vi "Teleop.vi"(10 "Match Info":T2={"Autonomous Elapsed Seconds"=0.0, "TeleOp Elapsed Seconds"=0.0, "Disabled Elapsed Seconds"=0.0, "Visited Autonomous"=FALSE, "Visited TeleOp"=FALSE, "Visited Disabled"=FALSE, "Autonomous Settings"={"Autonomous Style"=enum."Independent", "VI Refnum"=refnum}}, 11 "Call Context":T3) -> ()   [LabVIEW 2020]
doc: "This VI is called for each TeleOp packet received from the DS where the robot is not disabled. It is often used to read from the joysticks and update I/O or to update setpoints for timed control loops. It should complete and return within 20 milliseconds or it may miss DS packets."
uses:
  <vilib>/Rock Robotics/WPI/DriverStation/WPI_DriverStationDerivedRobotMode.ctl
  <vilib>/Rock Robotics/WPI/DriverStation/WPI_DriverStationMatch Info.ctl
  Shared Code/TypeDefs/ENUM_CMD_Mode Select.ctl
  Teleop Support/ENUM_Axes Select.ctl
  Teleop Support/ENUM_Button Select.ctl
  Systems/SwerveDrive/Cluster_CMD_ACT_Data.ctl
  Shared Code/TypeDefs/Cluster_CMD_Direction Data.ctl
  Shared Code/TypeDefs/Cluster_Module Velocity-Direction-Rotations.ctl
  Shared Code/TypeDefs/Level_Velocity plus-minus 1.ctl
  Shared Code/TypeDefs/Dial_Compase heading unit circle CCW positive.ctl
  Shared Code/TypeDefs/Cluster_X-Y.ctl
  Systems/PigeonIMU/Cluster_CMD_SEN_Data.ctl
  Systems/Tube Wheel/Cluster_CMD_ACT_Data.ctl
  Type Defs/ENUM_TubeWheel_Mode.ctl
  Type Defs/ENUM_Tube Wheel CMD Positions.ctl
  Systems/Angler/Cluster_CMD_ACT_Data.ctl
  Systems/Angler/ENUM_Input Mode.ctl
  Systems/Shooter/Cluster_CMD_ACT_Data.ctl
  Systems/Shooter/ENUM_Shooter_Mode.ctl
  Systems/Feeder/Cluster_CMD_ACT_Data.ctl
  Systems/Feeder/ENUM_CMD Mode.ctl
  Shared Code/TypeDefs/Cluster_High-Low.ctl
  8b3177bb-dc82-4863-aed5-aa104a122ccc.vi
  83fdd1ca-84e3-4cf5-86f5-8b3c56b849f5.vi
  <vilib>/Rock Robotics/Network Tables/NT Write Boolean.vi
  Systems/Game Controller/Global_SEN_Data Out.vi
  Systems/PigeonIMU/Global_CMD_SEN_Data In.vi
  Systems/Angler/Global_CMD_ACT_Data In.vi
  Systems/SwerveDrive/Global_CMD_ACT_Data In.vi
  Systems/Tube Wheel/Global_CMD_ACT_Data In.vi
  Systems/Shooter/Global_CMD_ACT_Data In.vi
  Systems/Feeder/Global_CMD_ACT_Data In.vi
  Systems/Game Controller/GameController_SEN.lvlib
  Systems/SwerveDrive/SwerveDrive_ACT_ts.lvlib
  Systems/PigeonIMU/PigeonIMU_SEN_ts.lvlib
  Systems/Tube Wheel/Tube Wheel_ACT.lvlib
  Systems/Angler/Angler_ACT.lvlib
  Systems/Shooter/Shooter_ACT.lvlib
  Systems/Feeder/Feeder_ACT.lvlib
panel:
  in  "MAx Traverse Speed FPS Out":dbl=5.0
  out "Drive Mode":T1
  out "shooter Speed Value":dbl
  in  "step value":dbl=200.0
  out "POV":i16
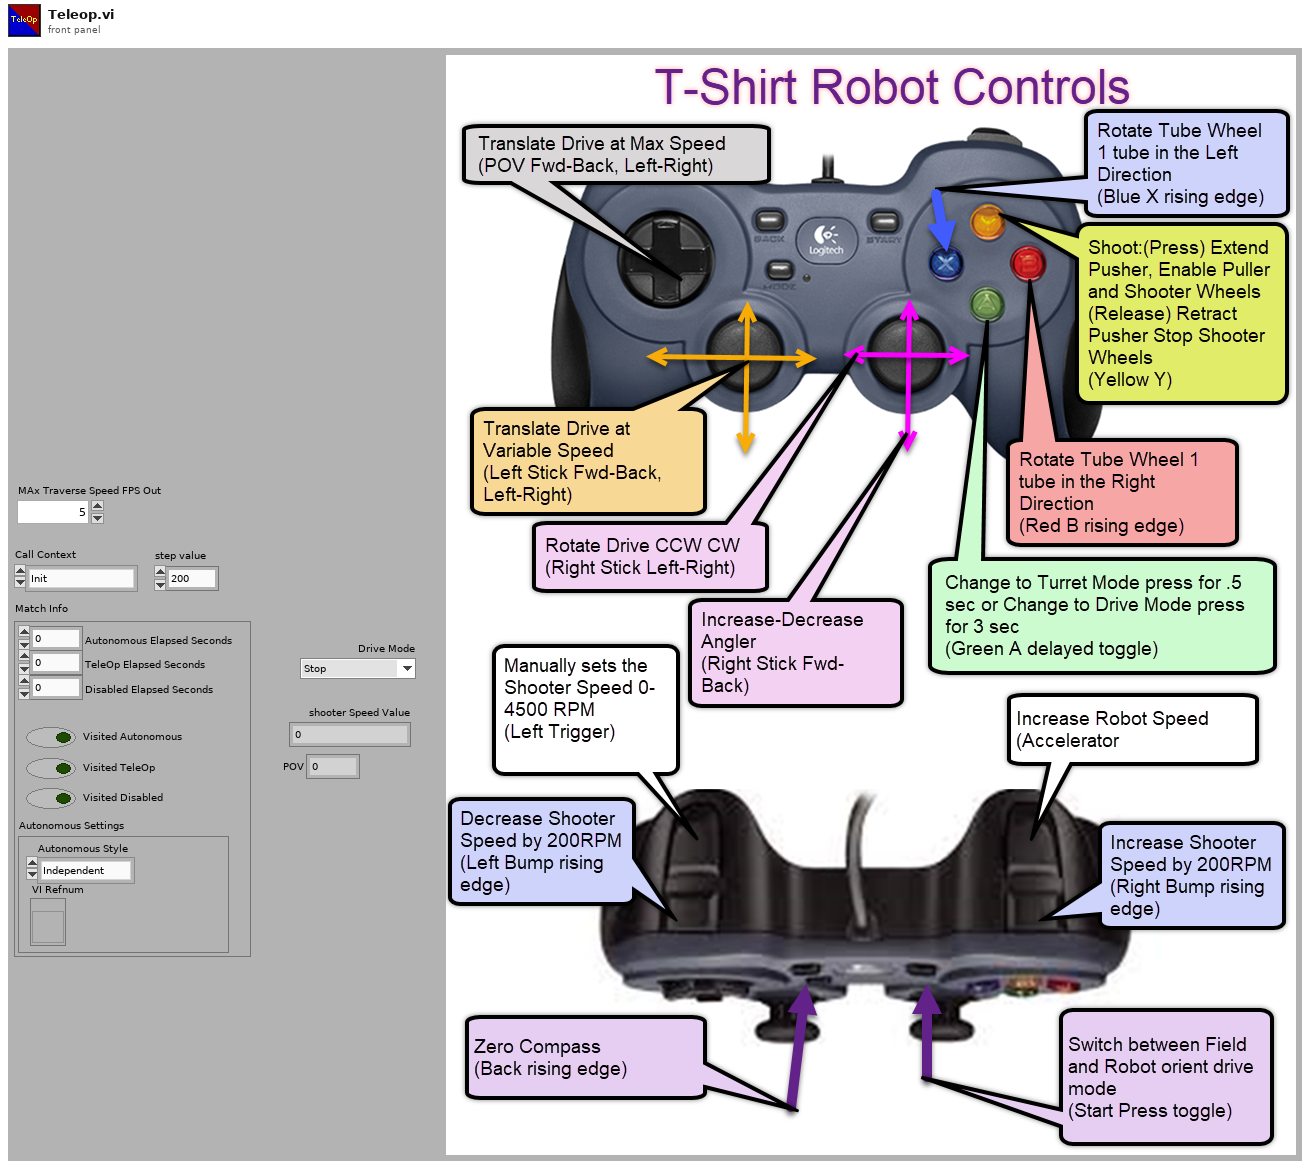
[diagram p1: front panel]
types:
  T1 = typedef "ENUM_CMD_Mode Select.ctl" = enum16{"Stop", "Move", "Turret Manual"}
  T2 = typedef "WPI_DriverStationMatch Info.ctl" = cluster{"Autonomous Elapsed Seconds":dbl, "TeleOp Elapsed Seconds":dbl, "Disabled Elapsed Seconds":dbl, "Visited Autonomous":bool, "Visited TeleOp":bool, "Visited Disabled":bool, "Autonomous Settings":cluster{"Autonomous Style":enum16{"Iterative", "Independent"}, "VI Refnum":refnum<vi>}}
  T3 = typedef "WPI_DriverStationDerivedRobotMode.ctl" = enum16{"Init", "Execute", "Stop"}
  T4 = typedef "ENUM_Axes Select.ctl" = enum16{"Left Stick Left (-1) Right (1)", "Left Stick Fwd (-1) Back(1)", "Left Trigger (0-1)", "Right Trigger (0-1)", "Right Stick Left(-1 Right (1)", "Right Stick Fwd(-1) Back (1)"}
  T5 = typedef "Cluster_High-Low.ctl" = cluster{"High":dbl, "Low":dbl}
  T6 = typedef "ENUM_Button Select.ctl" = enum16{"RightPad Green A", "RightPad Red B", "RightPad Blue X", "RightPad Yellow Y", "Left Bump", "Right Bump", "CenterPad Back", "CenterPad Start", "LeftStick Press", "RightStick Press"}
  T7 = typedef "Feeder_ACT.lvlib/Cluster_CMD_ACT_Data.ctl" = cluster{"Cmd Mode":T8, "Puller Speed (0-1":dbl}
  T8 = typedef "Feeder_ACT.lvlib/ENUM_CMD Mode.ctl" = enum16{"Stop", "Feed Pos 1", "Feed Pos 2", "Fead Full", "Back"}
  T9 = typedef "Shooter_ACT.lvlib/Cluster_CMD_ACT_Data.ctl" = cluster{"Mode":T10, "Speed Value":dbl}
  T10 = typedef "Shooter_ACT.lvlib/ENUM_Shooter_Mode.ctl" = enum16{"Stop", "Speed Percent", "Speed RPM"}
  T11 = typedef "Angler_ACT.lvlib/Cluster_CMD_ACT_Data.ctl" = cluster{"Mode":T12, "Speed -1 to 1":dbl, "Target Angle":dbl}
  T12 = typedef "Angler_ACT.lvlib/ENUM_Input Mode.ctl" = enum16{"Stop", "Speed", "Angle"}
  T13 = typedef "ENUM_Tube Wheel CMD Positions.ctl" = enum16{"Tube Red A", "Tube Black B", "Tube Red C", "Tube Black D", "Tube Red E", "Tube Black F"}
  T14 = typedef "Tube Wheel_ACT.lvlib/Cluster_CMD_ACT_Data.ctl" = cluster{"Mode":T15, "Target Tube Position":T13, "Motor speed (0-1)":dbl}
  T15 = typedef "ENUM_TubeWheel_Mode.ctl" = enum16{"Disabled", "Manual Motor", "Select Positon"}
  T16 = typedef "PigeonIMU_SEN_ts.lvlib/Cluster_CMD_SEN_Data.ctl" = cluster{"Reset":bool, "Disable":bool}
  T17 = typedef "Cluster_Module Velocity-Direction-Rotations.ctl" = cluster{"Velocity":T18, "Angle":T19, "Rotations Count":dbl}
  T18 = typedef "Level_Velocity plus-minus 1.ctl" = dbl
  T19 = typedef "Dial_Compase heading unit circle CCW positive.ctl" = dbl
  T20 = typedef "SwerveDrive_ACT_ts.lvlib/Cluster_CMD_ACT_Data.ctl" = cluster{"Mode":T1, "Direction":T21, "Orientation Robot(t) Field(f)":bool, "Max Translation Speed (ft/sec)":dbl, "Rotation Reduction 1-0":dbl, "Rotation Center from Robot Center":T22, "Auto Angle":T19, "Auto Target (ft)":dbl}
  T21 = typedef "Cluster_CMD_Direction Data.ctl" = cluster{"Traverse":T17, "Rotate(Yaw) CCW 1 CW -1":dbl}
  T22 = typedef "Cluster_X-Y.ctl" = cluster{"X":dbl, "Y":dbl}
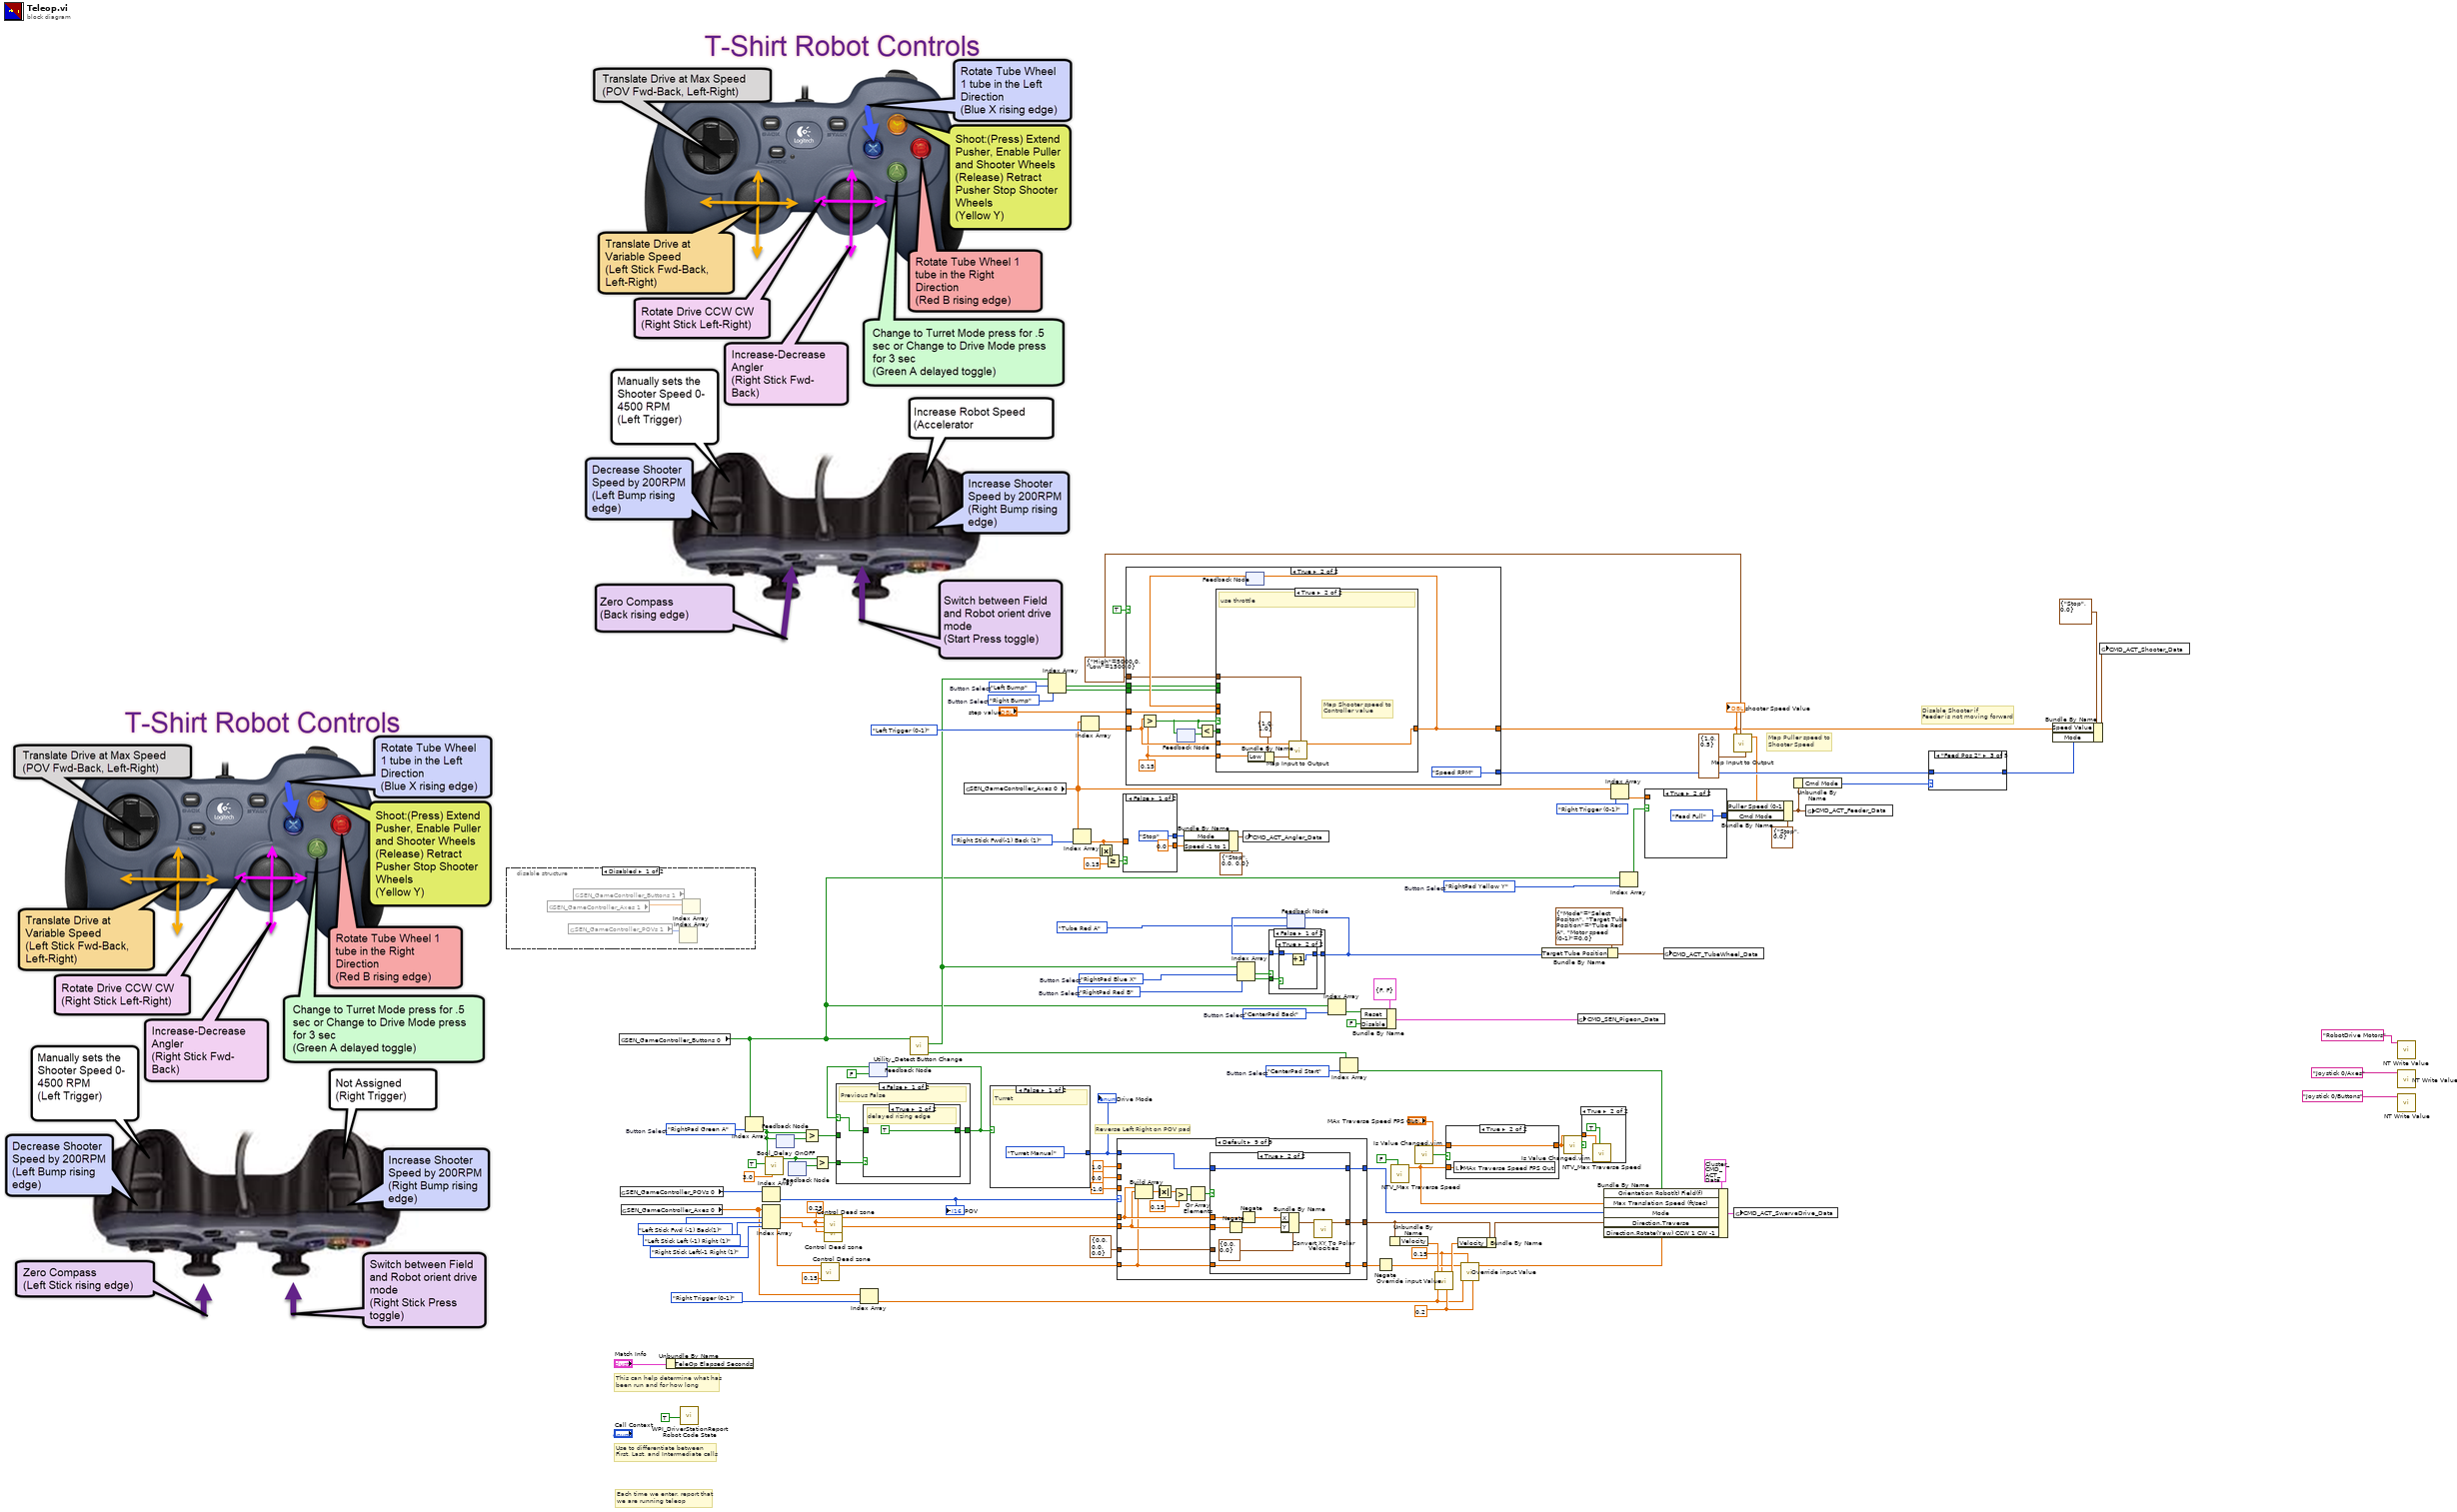
[diagram p0: block diagram]
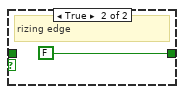
[diagram p6: hidden frame]
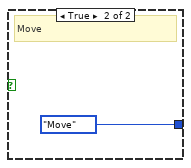
[diagram p7: hidden frame]
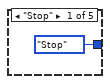
[diagram p8: hidden frame]
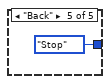
[diagram p11: hidden frame]
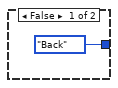
[diagram p12: hidden frame]
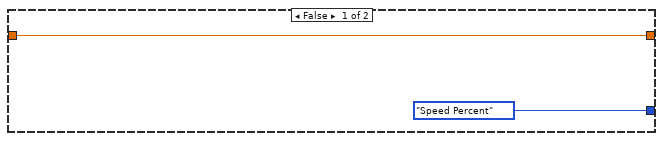
[diagram p13: hidden frame]
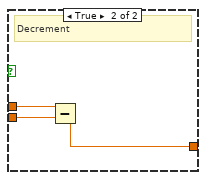
[diagram p15: hidden frame]
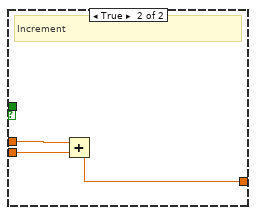
[diagram p16: hidden frame]
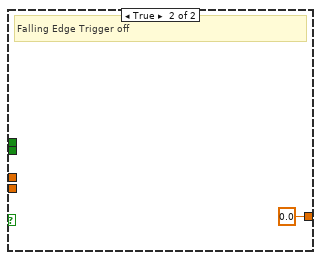
[diagram p17: hidden frame]
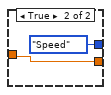
[diagram p18: hidden frame]
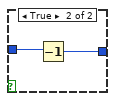
[diagram p20: hidden frame]
diagram:
  w8 = 0.2 ("lower limit")
  w9 = 0.15 ("upper limit")
  w40 = T5 {"High"=5000.0, "Low"=1500.0} ("Input Range")
  w48 = ENUM_Button_Select."RightPad Yellow Y"  # Button Select
  w56 = ENUM_Button_Select."Right Bump"  # Button Select
  w57 = ENUM_Button_Select."Left Bump"  # Button Select
  w72 = ENUM_Button_Select."RightPad Red B"  # Button Select
  w76 = ENUM_Button_Select."RightPad Blue X"  # Button Select
  w80 = ENUM_Button_Select."CenterPad Back"  # Button Select
  w87 = 0.25 ("y")
  w35 = ENUM_Button_Select."RightPad Green A"  # Button Select
  w85 = ENUM_Button_Select."CenterPad Start"  # Button Select
  # "Disable Shooter if\nFeeder is not moving forward"
  # "Map Puller speed to \nShooter Speed"
  # "Reverse Left Right on POV pad"
  # "Each time we enter, report that\nwe are running teleop"
  # "Use to differentiate between\nFirst, Last, and Intermediate calls"
  # "This can help determine what has\nbeen run and for how long"
  n1 = disable-structure shown="Disabled" {
    frame Disabled {
      n2 = global read "Global_SEN_Data Out.vi" "SEN_GameController_Axes 1"() -> (w111:dbl[])
      n3 = global read "Global_SEN_Data Out.vi" "SEN_GameController_POVs 1"() -> (w110:i16[])
      n4 = global read "Global_SEN_Data Out.vi" "SEN_GameController_Buttons 1"() -> ()  [unwired: 1 out]
      n5 = Index Array(array=w110) -> ()  [unwired: 1 in, 1 out]
      n6 = Index Array(array=w111) -> ()  [unwired: 1 in, 1 out]
    }
    frame Enabled {
    }
  }
  n7 = global read "Global_SEN_Data Out.vi" "SEN_GameController_Buttons 0"() -> (w20:bool[])
  n8 = global read "Global_SEN_Data Out.vi" "SEN_GameController_POVs 0"() -> (w104:i16[])
  n9 = global read "Global_SEN_Data Out.vi" "SEN_GameController_Axes 0"() -> (w18:dbl[])
  n10 = Unbundle By Name("Match Info") -> ()  [unwired: 1 out]
  n11 = call <vilib>:"WPI_DriverStationReport Robot Code State.vi"("TeleOp"=TRUE ("Autonomous")) -> ()  [unwired: 10 in, 1 out]
  n12 = Index Array(array=w20, index=w35) -> (element=w28:bool)
  n13 = Index Array(array=w18, index #1=ENUM_Axes_Select."Left Stick Fwd (-1) Back(1)" ("Axes Select"), index #2=ENUM_Axes_Select."Left Stick Left (-1) Right (1)" ("Axes Select"), index #3=ENUM_Axes_Select."Right Stick Left(-1 Right (1)" ("Axes Select")) -> (element #1=w93:dbl, element #2=w89:dbl, element #3=w88:dbl)
  n14 = Index Array(array=w104) -> (element=w101:i16)  [unwired: 1 in]
  "POV" <- w101
  n15 = call "Bool_Delay OnOFF.vi"("Delay Time(S)"=3.0, "Delay On(t) Off(f)"=TRUE, "Input"=w28) -> ("Output"=w29:bool)  [unwired: 7 in, 1 out]
  n16 = feedback #1() -> (w27:bool)  [unwired: 1 in]
  n17 = feedback-in #1(w28) -> ()
  n18 = feedback-in #2(w29) -> ()
  n19 = feedback #2() -> (w25:bool)  [unwired: 1 in]
  n20 = Greater?(x=w28, y=w27) -> (0:w26:bool)
  n21 = Greater?(x=w29, y=w25) -> (0:w24:bool)
  n22 = call "Control Dead zone.vi"("dead zone"=0.15 ("y"), "control Value"=w88) -> ("output Value"=w16:dbl)  [unwired: 9 in]
  n23 = call "Control Dead zone.vi"("dead zone"=w87, "control Value"=w93) -> ("output Value"=w92:dbl)  [unwired: 9 in]
  n24 = call "Control Dead zone.vi"("dead zone"=w87, "control Value"=w89) -> ("output Value"=w90:dbl)  [unwired: 9 in]
  n25 = Index Array(array=w18, index=ENUM_Axes_Select."Right Trigger (0-1)" ("Axes Select")) -> (element=w7:dbl)
  n26 = feedback #3(FALSE) -> (w33:bool)
  n27 = case shown="False" w33 {
    selector: w33 -> [w113 w118]
    tunnel: [w114 w119] -> w32
    tunnel: w26 -> [_ w117]
    tunnel: w24 -> [w112 _]
    frame False {
      # "Previous False"
      n28 = case shown="True" w112 {
        tunnel: [w115 TRUE] -> w114
        tunnel: w113 -> [w115 _]
        frame False {
        }
        frame True {
          # "delayed rizing edge"
        }
      }
    }
    frame True {
      # "Previous True"
      n29 = case shown="False" w117 {
        tunnel: [w120 FALSE] -> w119
        tunnel: w118 -> [w120 _]
        frame False {
          # "not Rizing"
        }
        frame True {
          # "rizing edge"
        }
      }
    }
  }
  n30 = feedback-in #3(w32) -> ()
  n31 = call "Utility_Detect Button Change.vi"("HW_Joystick_Buttons"=w20) -> ("Toggle On Rising Out"=w36:bool[], "Rising Out"=w49:bool[])  [unwired: 6 in, 3 out]
  n32 = global read "Global_SEN_Data Out.vi" "SEN_GameController_Axes 0"() -> (w46:dbl[])
  n33 = case shown="False" w32 {
    tunnel: [ENUM_CMD_Mode_Select."Turret Manual" ("Mode") ENUM_CMD_Mode_Select."Move" ("Mode")] -> w23
    frame False {
      # "Turret"
    }
    frame True {
      # "Move"
    }
  }
  "Drive Mode" <- w23
  n34 = Index Array(array=w49, index #1=w57, index #2=w56) -> (element #1=w52:bool, element #2=w54:bool)
  n35 = Index Array(array=w46, index=ENUM_Axes_Select."Right Stick Fwd(-1) Back (1)" ("Axes Select")) -> (element=w63:dbl)
  n36 = Index Array(array=w46, index=ENUM_Axes_Select."Left Trigger (0-1)" ("Axes Select")) -> (element=w55:dbl)
  n37 = Absolute Value(x=w63) -> (abs(x)=w66:dbl)
  n38 = Greater Or Equal?(x=w66, y=0.15) -> (x >= y?=w64:bool)
  n39 = case shown="Default" w101 {
    tunnel: 1.0 ("Direction.Travers Left 1 Right -1") -> [_ _ _ _ _ _ _ _ _]
    tunnel: 0.0 ("Direction.Travers Left 1 Right -1") -> [_ _ _ _ _ _ _ _ _]
    tunnel: -1.0 ("Direction.Travers Left 1 Right -1") -> [_ _ _ _ _ _ _ _ _]
    tunnel: w23 -> [w129 w135 w141 w147 w153 w159 w165 w171 w184]
    tunnel: [w129 w135 w141 w147 w153 w159 w165 w171 w183] -> w22
    tunnel: w92 -> [_ _ _ _ _ _ _ _ w181]
    tunnel: w90 -> [_ _ _ _ _ _ _ _ w180]
    tunnel: w16 -> [w128 w134 w140 w146 w152 w158 w164 w170 w179]
    tunnel: [w128 w134 w140 w146 w152 w158 w164 w170 w182] -> w94
    tunnel: T17 {"Velocity"=0.0, "Angle"=0.0, "Rotations Count"=0.0} ("Polar Out") -> [w127 w133 w139 w145 w151 w157 w163 w169 w173]
    tunnel: [w124 w130 w136 w142 w148 w154 w160 w166 w172] -> w14
    frame 0 {
      n40 = Bundle By Name(cluster=w127, "Velocity"=T18 1.0, "Angle"=T19 0.0) -> (w124:T17)
    }
    frame 45 {
      n41 = Bundle By Name(cluster=w133, "Velocity"=T18 1.0, "Angle"=T19 0.875) -> (w130:T17)
    }
    frame 90 {
      n42 = Bundle By Name(cluster=w139, "Velocity"=T18 1.0, "Angle"=T19 0.75) -> (w136:T17)
    }
    frame 135 {
      n43 = Bundle By Name(cluster=w145, "Velocity"=T18 1.0, "Angle"=T19 0.625) -> (w142:T17)
    }
    frame 180 {
      n44 = Bundle By Name(cluster=w151, "Velocity"=T18 1.0, "Angle"=T19 0.5) -> (w148:T17)
    }
    frame 225 {
      n45 = Bundle By Name(cluster=w157, "Velocity"=T18 1.0, "Angle"=T19 0.375) -> (w154:T17)
    }
    frame 270 {
      n46 = Bundle By Name(cluster=w163, "Velocity"=T18 1.0, "Angle"=T19 0.25) -> (w160:T17)
    }
    frame 315 {
      n47 = Bundle By Name(cluster=w169, "Velocity"=T18 1.0, "Angle"=T19 0.125) -> (w166:T17)
    }
    frame Default {
      n48 = Build Array(w181, w180, w179) -> (w178:dbl[])
      n49 = Absolute Value(x=w178) -> (abs(x)=w174:dbl[])
      n50 = Greater?(x=w174, y=0.15 ("upper limit")) -> (0:w176:bool[])
      n51 = Or Array Elements(Boolean array=w176) -> (logical OR=w175:bool)
      n52 = case shown="True" w175 {
        tunnel: w184 -> [_ w196]
        tunnel: [ENUM_CMD_Mode_Select."Stop" ("Mode") w196] -> w183
        tunnel: w181 -> [_ w198]
        tunnel: w180 -> [_ w197]
        tunnel: w179 -> [_ w195]
        tunnel: [0.0 ("f") w195] -> w182
        tunnel: w173 -> [w187 _]
        tunnel: [w188 w192] -> w172
        frame False {
          n53 = Bundle By Name(cluster=w187, "Velocity"=T18 0.0) -> (w188:T17)
        }
        frame True {
          n54 = Negate(x=w197) -> (-x=w191:dbl)
          n55 = Negate(x=w198) -> (-x=w190:dbl)
          n56 = Bundle By Name(cluster=T22 {"X"=0.0, "Y"=0.0} ("XY Velocities"), "X"=w190, "Y"=w191) -> (w194:T22)
          n57 = call "Convert XY To Polar Velocities.vi"("XY Velocities"=w194) -> ("Polar Out"=w192:T17)  [unwired: 10 in]
        }
      }
    }
  }
  n58 = case shown="False" w64 {
    tunnel: w63 -> [_ w201]
    tunnel: [ENUM_Input_Mode."Stop" ("Mode") ENUM_Input_Mode."Speed" ("Mode")] -> w62
    tunnel: [0.0 ("upper limit") w201] -> w61
    frame False {
    }
    frame True {
    }
  }
  n59 = case shown="True" TRUE {
    tunnel: w55 -> [w203 w216]
    tunnel: [w203 w215] -> w39
    tunnel: w54 -> [_ w213]
    tunnel: "step value" -> [_ w212]
    tunnel: w52 -> [_ w211]
    tunnel: [ENUM_Shooter_Mode."Speed Percent" ("Mode") ENUM_Shooter_Mode."Speed RPM" ("Mode")] -> w43
    tunnel: w40 -> [_ w205]
    frame False {
    }
    frame True {
      w209 = 0.15 ("y")
      n60 = Greater?(x=w216, y=w209) -> (0:w207:bool)
      n61 = feedback-in #4(w207) -> ()
      n62 = feedback #4() -> (w208:bool)  [unwired: 1 in]
      n63 = Less?(x=w207, y=w208) -> (x < y?=w206:bool)
      n64 = feedback #5() -> (w214:dbl)  [unwired: 1 in]
      n65 = case shown="True" w207 {
        tunnel: w216 -> [_ w245]
        tunnel: [w218 w244] -> w215
        tunnel: w214 -> [w221 _]
        tunnel: w213 -> [w222 _]
        tunnel: w212 -> [w220 _]
        tunnel: w211 -> [w219 _]
        tunnel: w209 -> [_ w241]
        tunnel: w206 -> [w217 _]
        tunnel: w205 -> [_ w240]
        frame False {
          # "Use step"
          n66 = case shown="False" w217 {
            tunnel: w222 -> [w227 _]
            tunnel: w221 -> [w226 _]
            tunnel: w220 -> [w225 _]
            tunnel: w219 -> [w224 _]
            tunnel: [w223 0.0] -> w218
            frame False {
              # "Not falling edge"
              n67 = case shown="False" w227 {
                tunnel: w226 -> [w231 w238]
                tunnel: w225 -> [w230 w237]
                tunnel: w224 -> [w228 _]
                tunnel: [w229 w236] -> w223
                frame False {
                  # "Don't increment"
                  n68 = case shown="False" w228 {
                    tunnel: w231 -> [w232 w235]
                    tunnel: w230 -> [_ w234]
                    tunnel: [w232 w233] -> w229
                    frame False {
                      # "Don't Decrement"
                    }
                    frame True {
                      # "Decrement"
                      n69 = Subtract(x=w235, y=w234) -> (x-y=w233:dbl)
                    }
                  }
                }
                frame True {
                  # "Increment"
                  n70 = Add(x=w238, y=w237) -> (x+y=w236:dbl)
                }
              }
            }
            frame True {
              # "Falling Edge Trigger off"
            }
          }
        }
        frame True {
          # "Map Shooter speed to \nController value"
          # "use throttle"
          n71 = Bundle By Name(cluster=T5 {"High"=1.0, "Low"=1.0} ("Input Range"), "Low"=w241) -> (w242:T5)
          n72 = call "Map Input to Output.vi"("output Range"=w240, "Input Range"=w242, "Input"=w245) -> ("output"=w244:dbl)  [unwired: 8 in]
        }
      }
      n73 = feedback-in #5(w215) -> ()
    }
  }
  "shooter Speed Value" <- w39
  n74 = Bundle By Name(cluster=T11 {"Mode"=enum."Stop", "Speed -1 to 1"=0.0, "Target Angle"=0.0} ("CMD_ACT_Angler_Data"), "Mode"=w62, "Speed -1 to 1"=w61) -> (w67:T11)
  n75 = Index Array(array=w49, index #1=w76, index #2=w72) -> (element #1=w75:bool, element #2=w71:bool)
  n76 = global write "Global_CMD_ACT_Data In.vi" "CMD_ACT_Angler_Data"(w67) -> ()
  n77 = feedback #6(ENUM_Tube_Wheel_CMD_Positions."Tube Red A" ("Target Tube Position")) -> (w74:T13)
  n78 = case shown="False" w75 {
    tunnel: w74 -> [w247 w253]
    tunnel: [w246 w252] -> w73
    tunnel: w71 -> [w248 _]
    frame False {
      n79 = case shown="True" w248 {
        tunnel: w247 -> [w249 w251]
        tunnel: [w249 w250] -> w246
        frame False {
        }
        frame True {
          n80 = Increment(x=w251) -> (x+1=w250:T13)
        }
      }
    }
    frame True {
      n81 = Decrement(x=w253) -> (x-1=w252:T13)
    }
  }
  n82 = feedback-in #6(w73) -> ()
  n83 = Index Array(array=w20, index=w80) -> (element=w81:bool)
  n84 = Index Array(array=w36, index=w85) -> (element=w84:bool)
  n85 = Bundle By Name(cluster=T16 {"Reset"=FALSE, "Disable"=FALSE} ("CMD_SEN_Pigeon_Data"), "Reset"=w81, "Disable"=FALSE) -> (w82:T16)
  n86 = Negate(x=w94) -> (-x=w11:dbl)
  n87 = Unbundle By Name(w14) -> ("Velocity"=w13:T18)
  n88 = call "NTV_Max Traverse Speed.vi"("Read(f) Write(t)"=FALSE) -> ("MAx Traverse Speed FPS Out"=w3:dbl)  [unwired: 10 in]
  n89 = call "Is Value Changed.vim"("value"=w3) -> ("changed or first call?"=w4:bool)
  n90 = call "Override input Value.vi"("Starting Override Value (0-1)"=w8, "Min Value To Overide (0-1)"=w9, "OverRide Value (0-1)"=w7, "Value In (0-1)"=w13) -> ("Value Out"=w12:T18)  [unwired: 7 in]
  n91 = case shown="True" w4 {
    tunnel: w3 -> [_ w256]
    tunnel: [w254 w255] -> w2
    tunnel: "MAx Traverse Speed FPS Out" -> [w254 w255]
    frame False {
    }
    frame True {
      n92 = local write "MAx Traverse Speed FPS Out"(w256) -> ()
    }
  }
  n93 = Bundle By Name(cluster=w14, "Velocity"=w12) -> (w15:T17)
  n94 = call "Override input Value.vi"("Starting Override Value (0-1)"=w8, "Min Value To Overide (0-1)"=w9, "OverRide Value (0-1)"=w7, "Value In (0-1)"=w11) -> ("Value Out"=w10:T18)  [unwired: 7 in]
  n95 = Bundle By Name(cluster=T14 {"Mode"=enum."Select Positon", "Target Tube Position"=enum."Tube Red A", "Motor speed (0-1)"=0.0} ("CMD_ACT_TubeWheel_Data"), "Target Tube Position"=w73) -> (w77:T14)
  n96 = call "Is Value Changed.vim"("value"=w2) -> ("changed or first call?"=w5:bool)
  n97 = global write "Global_CMD_SEN_Data In.vi" "CMD_SEN_Pigeon_Data"(w82) -> ()
  n98 = case shown="True" w5 {
    tunnel: w2 -> [_ w257]
    frame False {
    }
    frame True {
      n99 = call "NTV_Max Traverse Speed.vi"("Read(f) Write(t)"=TRUE, "MAx Tavers Speed FPS"=w257) -> ()  [unwired: 9 in, 1 out]
    }
  }
  n100 = Bundle By Name(cluster=T20 {"Mode"=enum."Stop", "Direction"={"Traverse"={"Velocity"=0.0, "Angle"=0.0, "Rotations Count"=0.0}, "Rotate(Yaw) CCW 1 CW -1"=0.0}, "Orientation Robot(t) Field(f)"=FALSE, "Max Translation Speed (ft/sec)"=0.0, "Rotation Reduction 1-0"=0.0, "Rotation Center from Robot Center"={"X"=0.0, "Y"=0.0}, "Auto Angle"=0.0, "Auto Target (ft)"=0.0} ("CMD_ACT_Template_Data"), "Orientation Robot(t) Field(f)"=w84, "Max Translation Speed (ft/sec)"=w3, "Mode"=w22, "Direction.Traverse"=w15, "Direction.Rotate(Yaw) CCW 1 CW -1"=w10) -> (w96:T20)
  n101 = Index Array(array=w46, index=ENUM_Axes_Select."Right Trigger (0-1)" ("Axes Select")) -> (element=w44:dbl)
  n102 = Index Array(array=w20, index=w48) -> (element=w47:bool)
  n103 = case shown="True" w47 {
    tunnel: [ENUM_CMD_Mode."Back" ("Cmd Mode") ENUM_CMD_Mode."Fead Full" ("Cmd Mode")] -> w21
    tunnel: w44 -> [_ _]
    frame False {
    }
    frame True {
    }
  }
  n104 = global write "Global_CMD_ACT_Data In.vi" "CMD_ACT_TubeWheel_Data"(w77) -> ()
  n105 = call "Map Input to Output.vi"("output Range"=T5 {"High"=1.0, "Low"=0.5}, "Input Range"=w40, "Input"=w39) -> ("output"=w37:dbl)  [unwired: 8 in]
  n106 = Bundle By Name(cluster=T7 {"Cmd Mode"=enum."Stop", "Puller Speed (0-1"=0.0} ("CMD_ACT_Feeder_Data"), "Puller Speed (0-1"=w37, "Cmd Mode"=w21) -> (w42:T7)
  n107 = global write "Global_CMD_ACT_Data In.vi" "CMD_ACT_SwerveDrive_Data"(w96) -> ()
  n108 = Unbundle By Name(w42) -> ("Cmd Mode"=w41:T8)
  n109 = global write "Global_CMD_ACT_Data In.vi" "CMD_ACT_Feeder_Data"(w42) -> ()
  n110 = case shown="\"Feed Pos 2\"" w41 {
    tunnel: w43 -> [_ w262 w263 w264 _]
    tunnel: [ENUM_Shooter_Mode."Stop" ("Mode") w262 w263 w264 ENUM_Shooter_Mode."Stop" ("Mode")] -> w19
    frame "Stop" {
    }
    frame "Feed Pos 1" {
    }
    frame "Feed Pos 2" {
    }
    frame "Fead Full" {
    }
    frame "Back" {
    }
  }
  n111 = Bundle By Name(cluster=T9 {"Mode"=enum."Stop", "Speed Value"=0.0} ("CMD_ACT_Shooter_Data"), "Speed Value"=w39, "Mode"=w19) -> (w59:T9)
  n112 = global write "Global_CMD_ACT_Data In.vi" "CMD_ACT_Shooter_Data"(w59) -> ()
  n113 = call-poly <vilib>:"NT Write Value.vi"("name"="RobotDrive Motors" ("Name")) -> ()  [unwired: 10 in, 1 out]
  n114 = call-poly <vilib>:"NT Write Value.vi"("name"="Joystick 0/Axes" ("Name")) -> ()  [unwired: 10 in, 1 out]
  n115 = call-poly <vilib>:"NT Write Value.vi"("name"="Joystick 0/Buttons" ("Name")) -> ()  [unwired: 10 in, 1 out]
